vi "LoadIconsIntoArray.vi"(7 "T- Name order/F-File order":bool, 8 "error in":errorcluster, 9 "Pattern":string="icons8*48.png", 10 "Path to PNG files":path=path "C:/Users/yoni/Downloads/file-circle-info.png", 11 "Name Order in":string[](array[string])=["add", "save", "print", "export", "reset", "view-details", "adjust", "zoom", "zoom-out", "zoom-to-actual-size", "hand-tool", "move", "histogram", "sine", "x-coordinate", "y-coordinate", "z-coordinate", "notification", "log", "grid", "filter-and-sort", "caliper", "comments", "triggering", "password"]) -> (0 "error out":errorcluster, 2 "Icon Sizes":i32[](array[numeric]), 4 "Icons out":picture[](array[picture]), 5 "Names out":string[](array[string])=["add", "save", "print", "export", "reset", "view-details", "adjust", "zoom", "zoom-out", "zoom-to-actual-size", "hand-tool", "move", "histogram", "sine", "x-coordinate", "y-coordinate", "z-coordinate", "notification", "log", "grid", "filter-and-sort", "caliper", "comments", "triggering", "password"], 6 "Raw 24-bit pixmaps":u32[][][](array[numeric]))   [LabVIEW 2023]
doc: "Load <strong>pattern</strong> picture files from <strong>PNG file path</strong> and (optionally) sort them according to <strong>Icon Names</strong> order. \n\n<strong>T- Name order/F- File order</strong> - Selects if outputs are set to Name of file order. \n<strong>Pattern</strong> - Pattern of the .png filenames to read from path. \n<strong>Path to PNG files</strong> - Path of the .png files to load. \n<strong>Names Order in</strong> - The name (the strings between outermost '-'s in the filenames) order of the requested image array. (Ignored if set to file order.)\n<strong>Icons out</strong> - The picture array of Icons output.\n<strong>Icon Sizes</strong> - The sizes of the icons' images that were read. \n<strong>Raw 24-bit pixmap</strong> - Output of the raw images data in 24-bit."
uses:
  <vilib>/picture/picture.llb/Draw True-Color Pixmap.vi
panel:
  out "FilePaths":path[](array[path])
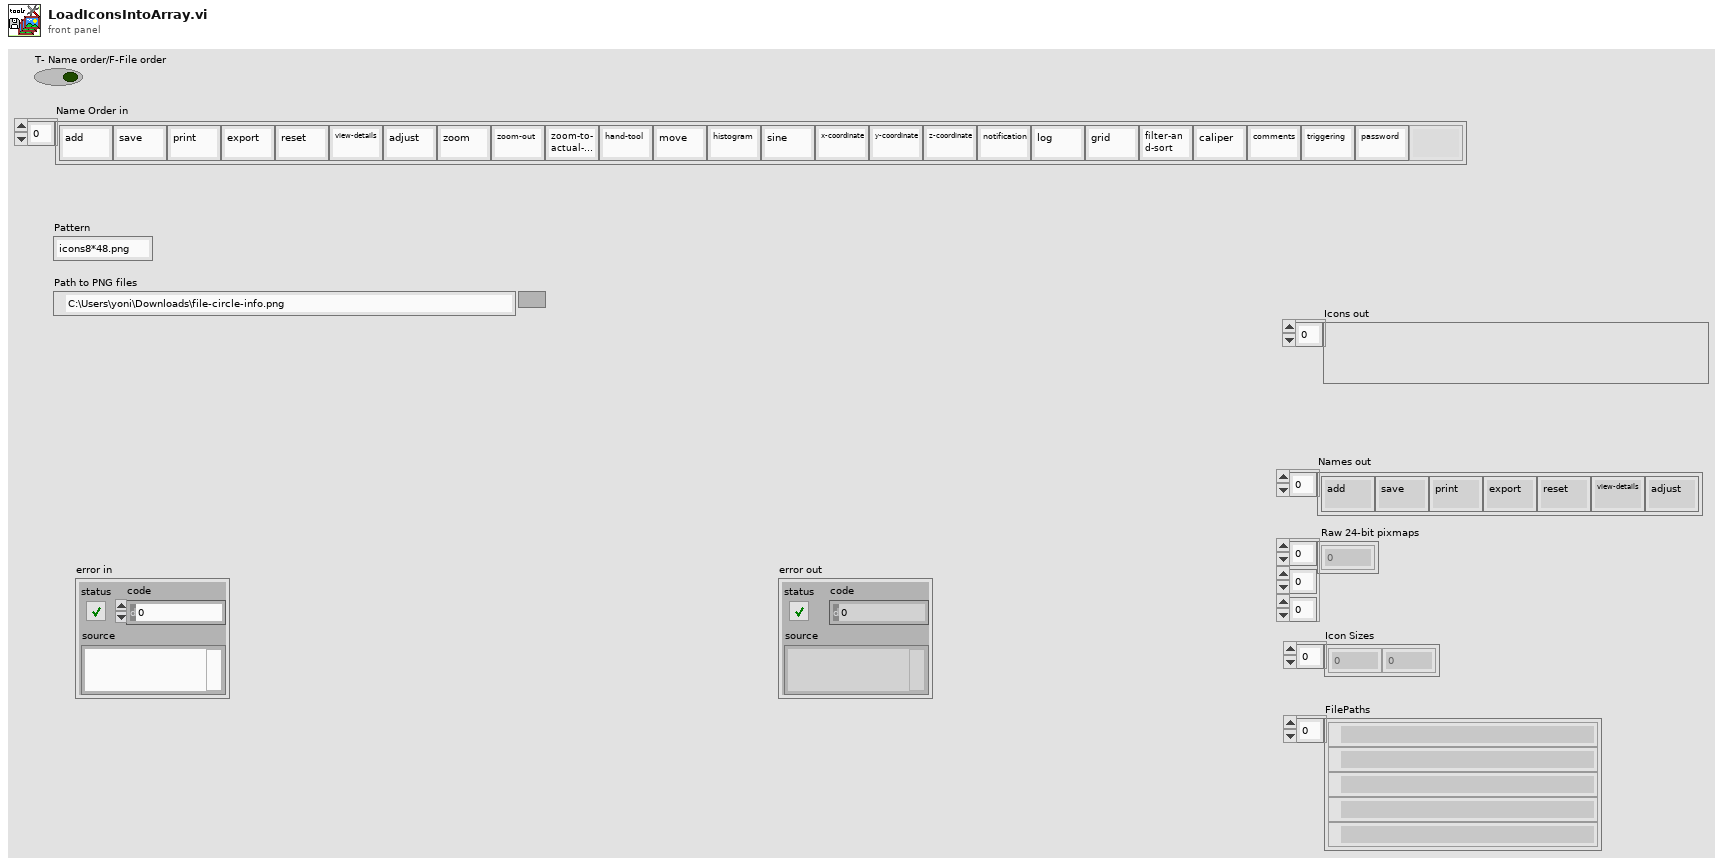
[diagram p1: front panel]
types:
  T1 = typedef "imagedata.ctl" = cluster{"image type":i32, "image depth":i32, "image":u8[], "mask":u8[], "colors":u32[], "Rectangle":cluster{"left":i16, "top":i16, "right":i16, "bottom":i16}}
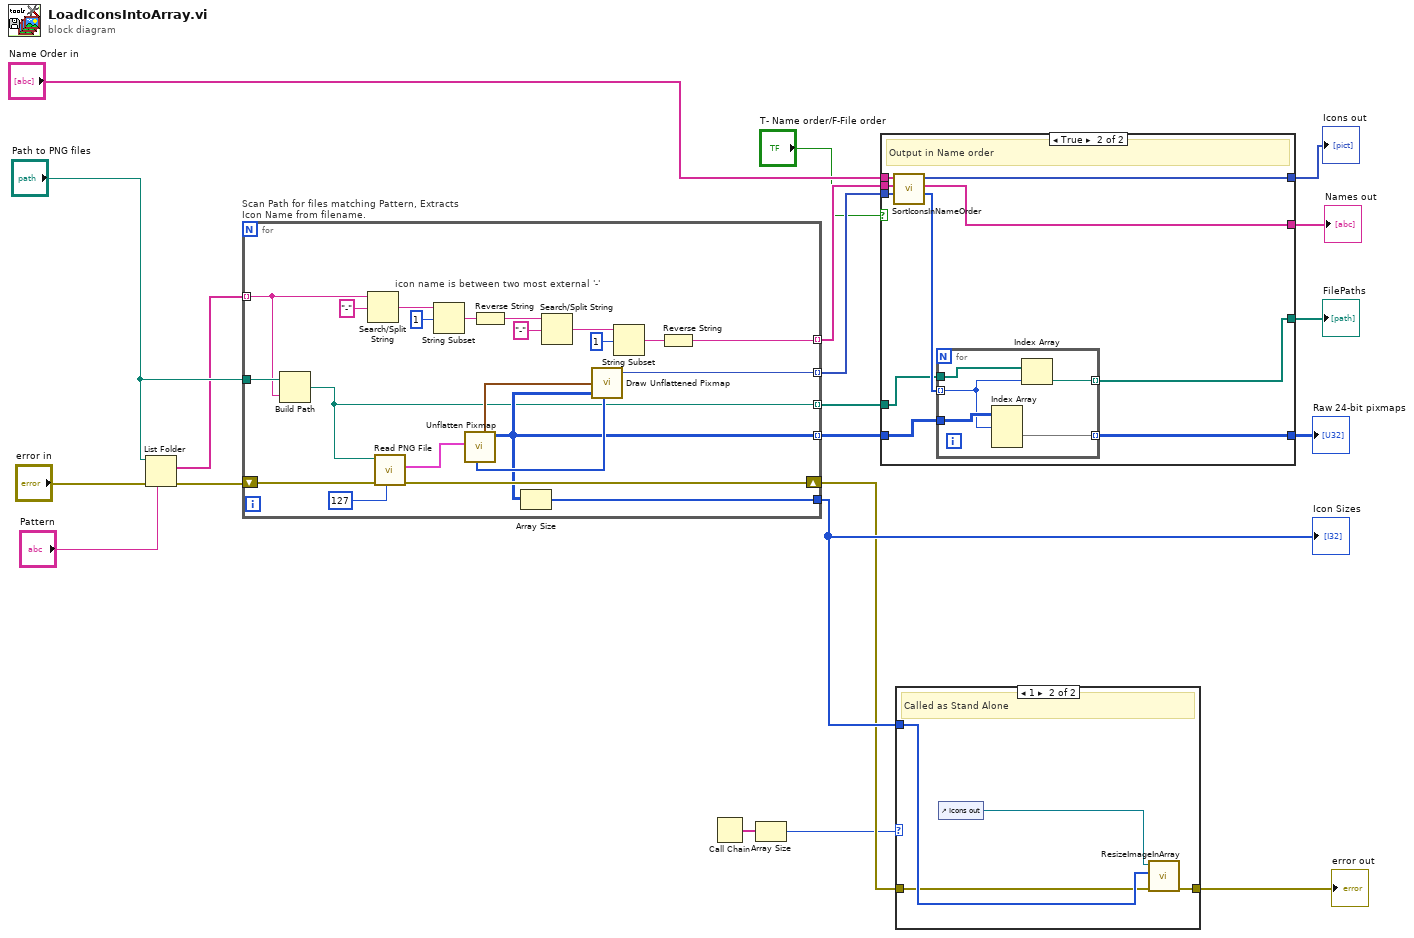
[diagram p0: block diagram]
diagram:
  n1 = List Folder(path="Path to PNG files", pattern="Pattern", error in="error in") -> (filenames=w8:string[], error out=w17:errorcluster)  [unwired: 1 in, 2 out]
  n2 = for "Scan Path for files matching Pattern, Extracts Icon Name from filename." {
    tunnel: [w42] -> w10 mode=indexing
    tunnel: "Path to PNG files" -> [w41]
    shift-right: [w36] -> w15
    shift-left: w17 -> [w37]
    tunnel: [w35] -> w16
    tunnel: [w23] -> w4 mode=indexing
    tunnel: w8 -> [w22] mode=indexing
    tunnel: [w33] -> w7 mode=indexing
    tunnel: [w21] -> w2 mode=indexing
    # "icon name is between two most external '-'"
    n3 = Build Path(base path=w41, name or relative path=w22) -> (appended path=w21:path)
    n4 = Search/Split String(string=w22, search string/char (-)="-") -> (match + rest of string=w29:string)  [unwired: 1 in, 2 out]
    n5 = call <vilib>:"Read PNG File.vi"("Transparency Thresh"=u8 127, "error in (no error)"=w37, "path to PNG file"=w21) -> ("error out"=w36:errorcluster, "image data"=w34:T1)  [unwired: 6 in, 1 out]
    n6 = String Subset(string=w29, offset (0)=1) -> (substring=w27:string)  [unwired: 1 in]
    n7 = call <vilib>:"Unflatten Pixmap.vi"("image data"=w34) -> ("24-bit pixmap"=w23:u32[][], "top left"=w39:cluster{"x":i16, "y":i16}, "mask"=w38:u8[])  [unwired: 4 in, 4 out]
    n8 = Reverse String(1:w27) -> (0:w31:string)
    n9 = Array Size(array=w23) -> (size(s)=w35:i32[])
    n10 = Search/Split String(string=w31, search string/char (-)="-") -> (match + rest of string=w25:string)  [unwired: 1 in, 2 out]
    n11 = call-poly <vilib>:"Draw Unflattened Pixmap.vi"("top left point(0, 0)"=w39, "data (RGB format)"=w23, "mask"=w38) -> ("new picture"=w42:picture)  [unwired: 6 in]
    n12 = String Subset(string=w25, offset (0)=1) -> (substring=w24:string)  [unwired: 1 in]
    n13 = Reverse String(1:w24) -> (0:w33:string)
  }
  "Icon Sizes" <- w16
  n14 = Call Chain() -> (call chain=w12:string[])
  n15 = Array Size(array=w12) -> (size(s)=w11:i32)
  n16 = case shown="True" "T- Name order/F-File order" {
    tunnel: [w46 w56] -> w20
    tunnel: w10 -> [w46 w55]
    tunnel: "Name Order in" -> [_ w54]
    tunnel: [w45 w53] -> w5
    tunnel: w7 -> [w45 w52]
    tunnel: w4 -> [w44 w51]
    tunnel: [w44 w49] -> w3
    tunnel: w2 -> [w43 w48]
    tunnel: [w43 w47] -> w1
    frame False {
      # "Output in file order"
    }
    frame True {
      # "Output in Name order"
      n17 = call "SortIconsInNameOrder.vi"("Icons File Order"=w55, "File Order"=w52, "Name Order"=w54) -> ("Order"=w50:i32[], "Icons names"=w53:string[], "Icons name order"=w56:picture[])  [unwired: 6 in]
      n18 = for {
        tunnel: w51 -> [w61]
        tunnel: w50 -> [w58] mode=indexing
        tunnel: [w60] -> w49 mode=indexing
        tunnel: w48 -> [w59]
        tunnel: [w57] -> w47 mode=indexing
        n19 = Index Array(array=w61, index (dim 0)=w58) -> (element=w60:u32[][])  [unwired: 2 in]
        n20 = Index Array(array=w59, index=w58) -> (element=w57:path)
      }
    }
  }
  "Icons out" <- w20
  "Names out" <- w5
  "Raw 24-bit pixmaps" <- w3
  "FilePaths" <- w1
  n21 = case shown="1" w11 {
    tunnel: w16 -> [_ w65]
    tunnel: w15 -> [w62 w63]
    tunnel: [w62 w64] -> w14
    frame Default {
      # "Called as subVI"
    }
    frame 1 {
      # "Called as Stand Alone"
      n22 = control-ref of="Icons out"() -> (w66:refnum<vi>)
      n23 = call "ResizeImageInArray.vi"("error in (no error)"=w63, "Draw Area Width/Height"=w65, "Array in"=w66) -> ("error out"=w64:errorcluster)  [unwired: 8 in]
    }
  }
  "error out" <- w14
